vi "OAT Linear Extrapolation.vi"(8 "extrapolation length":i32=2, 9 "modal length":i32=4, 10 "X[n]":dbl[](array[numeric]) format="%.2f") -> (1 "final":dbl[](array[numeric]) format="%.2f", 2 "X[n] out":dbl[](array[numeric]) format="%.2f", 3 "initail":dbl[](array[numeric]) format="%.2f")   [LabVIEW 2017, in "SoundVib_TachProcess.lvlib"]
uses:
  <vilib>/addons/Sound and Vibration/Order Analysis/Tach Process/SoundVib_TachProcess.lvlib
  <vilib>/Analysis/1siggen.llb/Ramp Pattern by Samples.vi
  <vilib>/Analysis/NI_AALPro.lvlib
  <vilib>/Analysis/NI_AALBase.lvlib
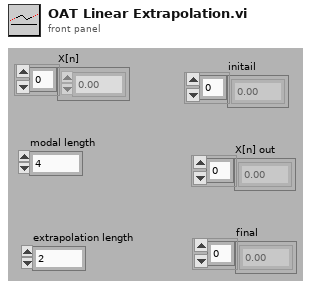
[diagram p1: front panel]
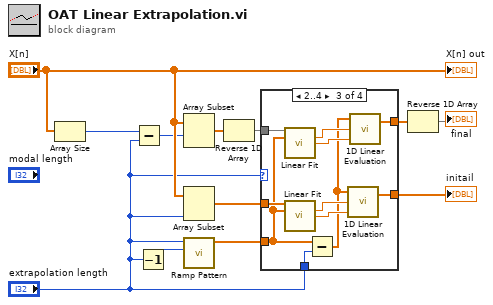
[diagram p0: block diagram]
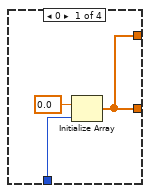
[diagram p2: hidden frame]
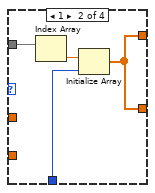
[diagram p3: hidden frame]
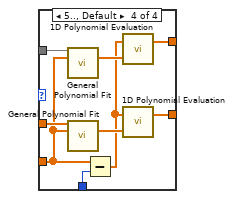
[diagram p4: hidden frame]
diagram:
  n1 = Array Size(array="X[n]") -> (size(s)=w4:i32)
  n2 = Subtract(x=w4, y="extrapolation length") -> (x-y=w11:i32)
  n3 = Decrement(x="extrapolation length") -> (x-1=w3:i32)
  n4 = Array Subset(array="X[n]", index=w11) -> (w10:dbl[])  [unwired: 1 in]
  n5 = Array Subset(array="X[n]", length="extrapolation length") -> (w7:dbl[])  [unwired: 1 in]
  n6 = call-poly <vilib>:"Ramp Pattern.vi"("end"=w3, "samples"="extrapolation length") -> ("Ramp Pattern"=w1:dbl[])  [unwired: 8 in, 1 out]
  n7 = Reverse 1D Array(array=w10) -> (reversed array=w8:dbl[])
  n8 = case shown="2..4" "extrapolation length" {
    tunnel: w8 -> [_ w19 w30 w39]
    tunnel: w7 -> [_ _ w29 w37]
    tunnel: [w13 w16 w25 w35] -> w6
    tunnel: [w13 w16 w26 w34] -> w5
    tunnel: w1 -> [_ _ w21 w33]
    tunnel: "extrapolation length" -> [w15 w17 w22 w32]
    frame 0 {
      n9 = Initialize Array(0.0 ("element"), w15) -> (w13:dbl[])
    }
    frame 1 {
      n10 = Index Array(array=w19) -> (element=w18:dbl)  [unwired: 1 in]
      n11 = Initialize Array(w18, w17) -> (w16:dbl[])
    }
    frame 2..4 {
      n12 = call <vilib>:"Linear Fit.vi"("Y"=w30, "X"=w21) -> ("slope"=w28:dbl, "intercept"=w27:dbl)  [unwired: 9 in, 3 out]
      n13 = call <vilib>:"Linear Fit.vi"("Y"=w29, "X"=w21) -> ("slope"=w24:dbl, "intercept"=w23:dbl)  [unwired: 9 in, 3 out]
      n14 = Subtract(x=w21, y=w22) -> (x-y=w20:dbl[])
      n15 = call <vilib>:"1D Linear Evaluation.vi"("offset"=w23, "scale"=w24, "X"=w20) -> ("Y[i]=X[i]*a+b"=w25:dbl[])  [unwired: 1 out]
      n16 = call <vilib>:"1D Linear Evaluation.vi"("offset"=w27, "scale"=w28, "X"=w20) -> ("Y[i]=X[i]*a+b"=w26:dbl[])  [unwired: 1 out]
    }
    frame 5.., Default {
      n17 = call <vilib>:"General Polynomial Fit.vi"("Y"=w39, "X"=w33) -> ("Polynomial Coefficients"=w38:dbl[])  [unwired: 10 in, 3 out]
      n18 = call <vilib>:"General Polynomial Fit.vi"("Y"=w37, "X"=w33) -> ("Polynomial Coefficients"=w36:dbl[])  [unwired: 10 in, 3 out]
      n19 = Subtract(x=w33, y=w32) -> (x-y=w31:dbl[])
      n20 = call <vilib>:"1D Polynomial Evaluation.vi"("Coefficients: a"=w38, "X"=w31) -> ("Y"=w34:dbl[])  [unwired: 1 out]
      n21 = call <vilib>:"1D Polynomial Evaluation.vi"("Coefficients: a"=w36, "X"=w31) -> ("Y"=w35:dbl[])  [unwired: 1 out]
    }
  }
  "initail" <- w6
  n22 = Reverse 1D Array(array=w5) -> (reversed array=→"final":dbl[])
  "X[n] out" <- "X[n]"
